vi "제목없음 2.vi"() -> ()   [LabVIEW 2014]
panel:
  in  "불리언":bool
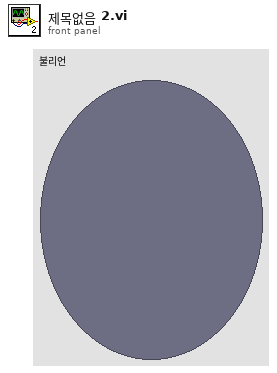
[diagram p1: front panel]
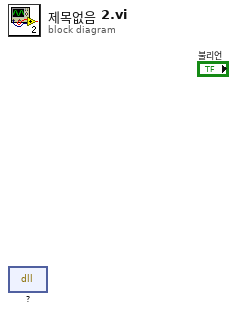
[diagram p0: block diagram]
diagram:
  n1 = dll-call lib="?" fn="?"() -> ()  [unwired: 4 in, 2 out]
